vi "global_state_notifier.vi"() -> (0 "error out":errorcluster, 3 "GLOBAL STATE":refnum<notifier>)   [LabVIEW 2013]
uses:
  main_machine/type_defs/mm_states.ctl
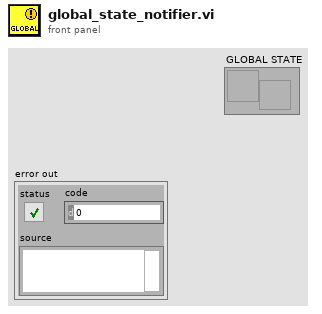
[diagram p1: front panel]
types:
  T1 = typedef "mm_states.ctl" = enum16{"STARTUP", "WAIT FOR COMMAND", "INITIALIZE INSTRUMENT", "FIND FCS FILE ", "START EXPERIMENT", "WAIT TO SAMPLE ", "DILUTE", "TAKE SAMPLE ", "EXIT"}
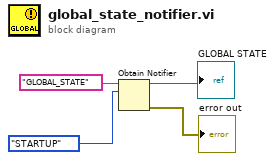
[diagram p0: block diagram]
diagram:
  n1 = Obtain Notifier(name (unnamed)="GLOBAL_STATE", notification data type=mm_states."STARTUP" ("element")) -> (notifier out=→"GLOBAL STATE":refnum<notifier>, error out=→"error out":errorcluster)  [unwired: 2 in, 1 out]
